vi "Tic Tac Toe.vi"() -> ()   [LabVIEW 2015]
panel:
  in  "o":u16(ring)
  in  "x":u16(ring)
  in  "Array":u16[][](array[ring])
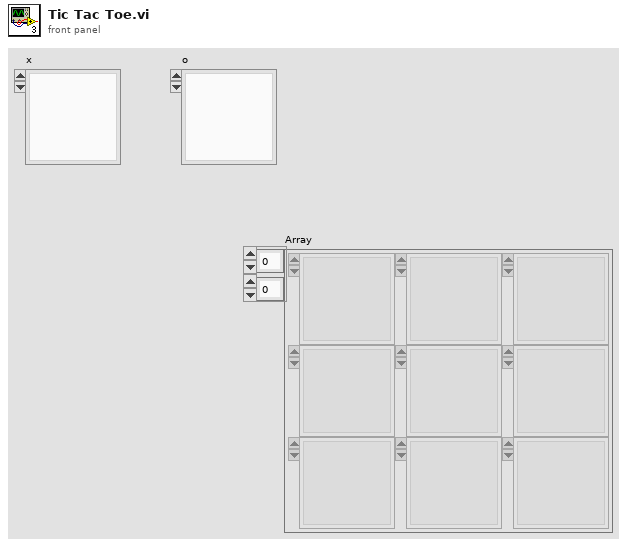
[diagram p1: front panel]
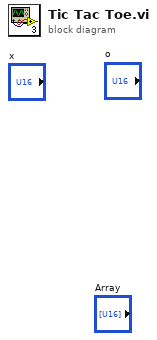
[diagram p0: block diagram]
diagram:
